vi "PXI-Set AI Gains.vi"(7 "AI Tasks":T1[](array[typedef])=[{"Task name"="AI01", "Task"="", "Dual-channel task?"=FALSE, "Regenerate?"=FALSE, "Clear?"=FALSE}], 11 "error in (no error)":errorcluster) -> (8 "AI Tasks out":T1[](array[typedef])=[{"Task name"="AI01", "Task"="", "Dual-channel task?"=FALSE, "Regenerate?"=FALSE, "Clear?"=FALSE}], 15 "error out":errorcluster)   [LabVIEW 2020]
uses:
  Type Defs/Task Struct.ctl
  PXI Globals.vi
  <resource>/objmgr/daqmx.rc
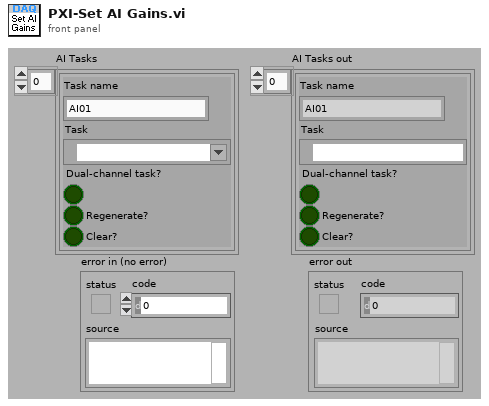
[diagram p1: front panel]
types:
  T1 = typedef "Task Struct.ctl" = cluster{"Task name":string, "Task":refnum<k21>, "Dual-channel task?":bool, "Regenerate?":bool, "Clear?":bool}
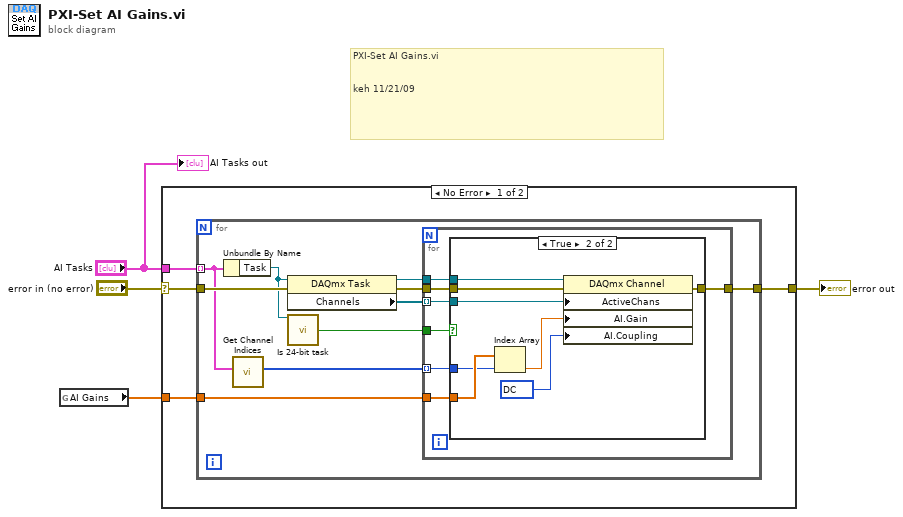
[diagram p0: block diagram]
diagram:
  # "PXI-Set AI Gains.vi\n\n\nkeh 11/21/09"
  n1 = global read "PXI Globals.vi" "AI Gains"() -> (w2:dbl[])
  n2 = case shown="No Error" "error in (no error)" {
    selector: "error in (no error)" -> [w7 w35]
    tunnel: [w6 w35] -> w3
    tunnel: "AI Tasks" -> [w8 _]
    tunnel: w2 -> [w5 _]
    frame No Error {
      n3 = for {
        tunnel: w8 -> [w13] mode=indexing
        tunnel: w7 -> [w18]
        tunnel: [w15] -> w6
        tunnel: w5 -> [w14]
        n4 = Unbundle By Name(w13) -> ("Task"=w9:refnum<k21>)
        n5 = call "Get Channel Indices.vi"("Task Structure"=w13) -> ("Channel Indices"=w12:i32[])  [unwired: 10 in]
        n6 = property class="DAQmx Task"(reference=w9, error in=w18) -> (reference out=w11:refnum<k21>, error out=w17:errorcluster, "Channels"=w16:refnum<k21>[])
        n7 = call "Is 24-bit task.vi"("task"=w9) -> ("is 24bit?"=w10:bool)  [unwired: 9 in, 5 out]
        n8 = for {
          tunnel: w10 -> [w25]
          tunnel: w17 -> [w24]
          tunnel: w16 -> [w23] mode=indexing
          tunnel: [w22] -> w15
          tunnel: w14 -> [w21]
          tunnel: w12 -> [w20] mode=indexing
          tunnel: w11 -> [w19]
          n9 = case shown="True" w25 {
            tunnel: w24 -> [w26 w34]
            tunnel: w23 -> [_ w30]
            tunnel: [w26 w33] -> w22
            tunnel: w21 -> [_ w32]
            tunnel: w20 -> [_ w31]
            tunnel: w19 -> [_ w29]
            frame False {
            }
            frame True {
              w27 = 10050 items=["AC"=10045, "DC"=10050, "GND"=10066] ("AI.Coupling")
              n10 = Index Array(array=w32, index=w31) -> (element=w28:dbl)
              n11 = property class="DAQmx Channel"(reference=w29, error in=w34, "ActiveChans"=w30, "AI.Gain"=w28, "AI.Coupling"=w27) -> (error out=w33:errorcluster)  [unwired: 1 out]
            }
          }
        }
      }
    }
    frame Error {
    }
  }
  "error out" <- w3
  "AI Tasks out" <- "AI Tasks"
